vi "(FPGA)_PIDXYZ_laserPID)_COMtemp_vec_1.vi"() -> ()   [LabVIEW 2018]
doc: "This VI will read single point values from 4 channels of a R Series board at a specified rate."
uses:
  <vilib>/rvi/Emulation/niFpgaGetClockAttributes.vi
  <vilib>/rvi/Emulation/niFpgaSctlEmulationGetInTimedLoop.vi
  <vilib>/rvi/Emulation/niFpgaEmulationReportErrorSimple.vi
  <vilib>/rvi/eio/common/nirviEmuTemplateMethod_errors.vi
  <vilib>/rvi/Emulation/niFpgaProcessEmulError.vi
  <vilib>/rvi/Emulation/niFpgaCriticalErrorInLSC.vi
  <vilib>/rvi/Memory/Memory_Emulation/nirvimemoryFastEmulation.vi
  <vilib>/rvi/Memory/Memory_Emulation/nirvimemoryEmulation.vi
  <vilib>/rvi/Emulation/niFpgaEmulationIsFPGAContextNoSignature.vi
  <vilib>/rvi/DataTransferAndStorage/Container/Common/niFpgaContainerGetUniqueNameForEmu.vi
  <vilib>/rvi/errors/nirviReportUnexpectedCaseInternalError (U32).vi
  <vilib>/rvi/Memory/Memory_Emulation/niFpgaMemoryEmulationCacheClearOnFirstRun.vi
  <vilib>/rvi/Memory/Memory_Emulation/nirvimemoryEmulationManagerCache_MakeExclusive.vi
  <vilib>/rvi/Memory/Memory_Emulation/niFpgaMemoryEmulationValidateCache.vi
  <vilib>/rvi/Memory/Memory_Emulation/nirvimemoryEmulationManagerCache_InsertValue.vi
  <vilib>/Utility/error.llb/Clear Errors.vi
  <vilib>/rvi/Memory/Memory_Emulation/nirvimemoryEmulationManagerCache_ReleaseExclusive.vi
  <vilib>/rvi/Memory/Memory_Emulation/nirvimemoryEmulationManagerCache_GetValue.vi
  <vilib>/rvi/Memory/Memory_Emulation/nirvimemoryEmulationManagerCache_SetValue.vi
  <vilib>/rvi/Emulation/niFpgaSctlEmulationResourceMgr.vi
  <vilib>/eio/EIONode/EIONode.xnode
  <vilib>/rvi/DataTransferAndStorage/Container/XNode/niFpgaContainer.xnode
  <vilib>/rvi/FXPMathLib/FxpInterpret/XNode/nifxpmath_Interpret.xnode
panel:
  in  "Amplitude AO7":fxp<+/-,64,32>
  in  "Amplitude AO6":fxp<+/-,64,32>
  in  "Amplitude AO5":fxp<+/-,64,32>
  in  "Amplitude AO4":fxp<+/-,64,32>
  in  "phase offset AO7":fxp<+,32,0>
  in  "reset AO7":bool
  in  "frequency AO7":fxp<+,32,0>=0.0002500000409781933
  in  "phase offset AO6":fxp<+,32,0>
  in  "reset AO6":bool
  in  "frequency AO6":fxp<+,32,0>=0.0002500000409781933
  in  "phase offset AO5":fxp<+,32,0>
  in  "reset AO5":bool
  in  "frequency AO5":fxp<+,32,0>=0.0002500000409781933
  in  "phase offset AO4":fxp<+,32,0>
  in  "reset AO4":bool
  in  "frequency AO4":fxp<+,32,0>=0.0002500000409781933
  in  "stop":bool
  in  "Notch coeff y 2":i32[](array[numeric])=[-1060332860, 1067037342, -2129863576]
  in  "Notch coeff y 1":i32[](array[numeric])=[-1060332860, 1067037342, -2129863576]
  in  "Notch coeff x":i32[](array[numeric])=[-1060332860, 1067037342, -2129863576]
  out "accum out z2":fxp<+/-,37,37>
  out "accurm reset z2":bool
  out "accum out z1":fxp<+/-,37,37>
  out "accum reset z1":bool
  in  "Reset x accum":bool
  in  "Reset y accum":bool
  in  "Reset z accum":bool
  out "master y":bool
  out "master x":bool
  in  "No_integral_gain":bool=TRUE
  in  "Y_emergency_threshould":i16
  in  "X_emergency_threshould":i16
  in  "Big Number":sgl
  in  "Amplitude_sine_EOM":sgl
  in  "eom sine frequency (periods/tick)":fxp<+,32,0>=0.0002500000409781933
  in  "pz?":bool
  out "pg Z mod":fxp<+/-,24,12>
  in  "pg Z":fxp<+/-,24,12>
  in  "amplitude":i16=8192
  in  "offset":i16=8192
  out "Trigger for COM out":i16 caption="square wave out"
  out "dgz mod":fxp<+/-,24,12>
  in  "activate COMz":bool
  in  "dg Z":fxp<+/-,24,12>
  in  "activate COMy":bool
  out "dgy mod":fxp<+/-,24,12>
  in  "dg Y":fxp<+/-,24,12>
  out "dgx mod":fxp<+/-,24,12>
  in  "activate COMx":bool
  in  "dg X":fxp<+/-,24,12>
  in  "duty cycle (periods)":fxp<+,32,0>=0.5
  in  "frequency (periods/tick)":fxp<+,32,0>=0.00390625
  in  "final filter coeff X before":i32[](array[numeric])=[-955995012, 2025731616, 1001305, -1023351008, 2092954700, 1034533]
  in  "final filter coeff X":i32[](array[numeric])=[-955995012, 2025731616, 1001305, -1023351008, 2092954700, 1034533]
  in  "final filter coeff Y before":i32[](array[numeric])=[-955995012, 2025731616, 1001305, -1023351008, 2092954700, 1034533]
  in  "final filter coeff Y":i32[](array[numeric])=[-955995012, 2025731616, 1001305, -1023351008, 2092954700, 1034533]
  in  "final filter coeff Z":i32[](array[numeric])=[-955995012, 2025731616, 1001305, -1023351008, 2092954700, 1034533]
  in  "final filter coeff Z before":i32[](array[numeric])=[-955995012, 2025731616, 1001305, -1023351008, 2092954700, 1034533]
  in  "LP Coeff Z before":i32[](array[numeric])=[1008310688, 32715568]
  in  "LP Coeff Z":i32[](array[numeric])=[1008310688, 32715568]
  in  "LP Coeff X":i32[](array[numeric])=[1008310688, 32715568]
  in  "LP Coeff X before":i32[](array[numeric])=[1008310688, 32715568]
  in  "LP Coeff Y before":i32[](array[numeric])=[1008310688, 32715568]
  in  "LP Coeff Y":i32[](array[numeric])=[1008310688, 32715568]
  in  "Upper lim Z before":fxp<+/-,16,16>
  in  "Lower lim Z before":fxp<+/-,16,16>
  in  "Upper lim Y before":fxp<+/-,16,16>
  in  "Lower lim Y before":fxp<+/-,16,16>
  in  "Upper lim X before":fxp<+/-,16,16>
  in  "Lower lim X before":fxp<+/-,16,16>
  in  "HP coeff band X before":i32[](array[numeric])=[-850883994, 1909449570, 958518847, -975456236, 2033039520, 1020559395]
  in  "LP Coeff band X before":i32[](array[numeric])=[-955995012, 2025731616, 1001305, -1023351008, 2092954700, 1034533]
  in  "LP Coeff band X":i32[](array[numeric])=[-955995012, 2025731616, 1001305, -1023351008, 2092954700, 1034533]
  in  "HP Coeff band X":i32[](array[numeric])=[-850883994, 1909449570, 958518847, -975456236, 2033039520, 1020559395]
  in  "dg band X before":fxp<+/-,24,12>
  in  "dg band X":fxp<+/-,24,12>
  in  "HP Coeff X before":i32[](array[numeric])=[946630756, 1010186290]
  in  "HP Coeff X":i32[](array[numeric])=[946630756, 1010186290]
  in  "Use X PID before":bool
  out "AI X before chamber plot":i16
  in  "X before Setpoint":i16
  out "tot_fb X plot":i16
  out "fb X before chamber plot":i16
  in  "DC offset X":i16
  in  "pg X before":fxp<+/-,24,12>
  in  "ig X before":fxp<+/-,24,-4>
  in  "dg X before":fxp<+/-,24,12>
  out "fb X plot":i16
  in  "ig X":fxp<+/-,24,-4>
  in  "Lower lim X":fxp<+/-,16,16>
  in  "Upper lim X":fxp<+/-,16,16>
  in  "pg X":fxp<+/-,24,12>
  out "AI X plot":i16
  in  "X Setpoint":i16
  in  "HP coeff band Y before":i32[](array[numeric])=[-850883994, 1909449570, 958518847, -975456236, 2033039520, 1020559395]
  in  "LP Coeff band Y before":i32[](array[numeric])=[-955995012, 2025731616, 1001305, -1023351008, 2092954700, 1034533]
  in  "LP Coeff band Y":i32[](array[numeric])=[-955995012, 2025731616, 1001305, -1023351008, 2092954700, 1034533]
  in  "HP Coeff band Y":i32[](array[numeric])=[-850883994, 1909449570, 958518847, -975456236, 2033039520, 1020559395]
  in  "dg band Y before":fxp<+/-,24,12>
  in  "dg band Y":fxp<+/-,24,12>
  in  "HP Coeff Y before":i32[](array[numeric])=[946630756, 1010186290]
  in  "HP Coeff Y":i32[](array[numeric])=[946630756, 1010186290]
  in  "Use Y PID before":bool
  out "AI Y before chamber plot":i16
  in  "Y before Setpoint":i16
  out "tot_fb Y plot":i16
  out "fb Y before chamber plot":i16
  in  "DC offset Y":i16
  in  "pg Y before":fxp<+/-,24,12>
  in  "ig Y before":fxp<+/-,24,-4>
  in  "dg Y before":fxp<+/-,24,12>
  out "fb Y plot":i16
  in  "ig Y":fxp<+/-,24,-4>
  in  "Lower lim Y":fxp<+/-,16,16>
  in  "Upper lim Y":fxp<+/-,16,16>
  in  "pg Y":fxp<+/-,24,12>
  out "AI Y plot":i16
  in  "Y Setpoint":i16
  in  "EOM_offset":i16
  in  "EOM_seed":u32=4294967295 caption="seed"
  in  "EOM reset":bool caption="reset"
  in  "EOM_threshold":i16
  in  "EOM_amplitude":i16
  in  "HP coeff band Z before":i32[](array[numeric])=[-850883994, 1909449570, 958518847, -975456236, 2033039520, 1020559395]
  in  "LP Coeff band Z before":i32[](array[numeric])=[-955995012, 2025731616, 1001305, -1023351008, 2092954700, 1034533]
  in  "LP Coeff band Z":i32[](array[numeric])=[-955995012, 2025731616, 1001305, -1023351008, 2092954700, 1034533]
  in  "HP Coeff band Z":i32[](array[numeric])=[-850883994, 1909449570, 958518847, -975456236, 2033039520, 1020559395]
  in  "dg band Z before":fxp<+/-,24,12>
  in  "dg band Z":fxp<+/-,24,12>
  in  "data_buffer3":i16
  in  "Arb gain (ch2)":fxp<+/-,24,12>=0.5 caption="RMS"
  in  "HP Coeff Z before":i32[](array[numeric])=[946630756, 1010186290]
  in  "HP Coeff Z":i32[](array[numeric])=[946630756, 1010186290]
  in  "Use Z PID before":bool
  out "AI Z before chamber plot":i16
  in  "Z before Setpoint":i16
  out "tot_fb Z plot":i16
  out "fb Z before chamber plot":i16
  in  "DC offset Z":i16
  in  "pg Z before":fxp<+/-,24,12>
  in  "ig Z before":fxp<+/-,24,-4>
  in  "dg Z before":fxp<+/-,24,12>
  out "fb Z plot":i16
  in  "ig Z":fxp<+/-,24,-4>
  out "written_address":u32
  in  "ready_to_write":bool
  in  "Arb steps per cycle":u16
  in  "data_buffer2":i16
  in  "data_buffer_1":i16
  in  "write_address":u16
  in  "Arb gain (ch1)":fxp<+/-,24,12>=0.5 caption="RMS"
  in  "Arb gain (ch0)":fxp<+/-,24,12>=0.5 caption="RMS"
  in  "Lower lim Z":fxp<+/-,16,16>
  in  "Upper lim Z":fxp<+/-,16,16>
  out "AI Z plot":i16
  in  "Z Setpoint":i16
  in  "Count(uSec)":u32
  out "FPGA Error Out":errorcluster
  in  "Stop":bool
  # "test"
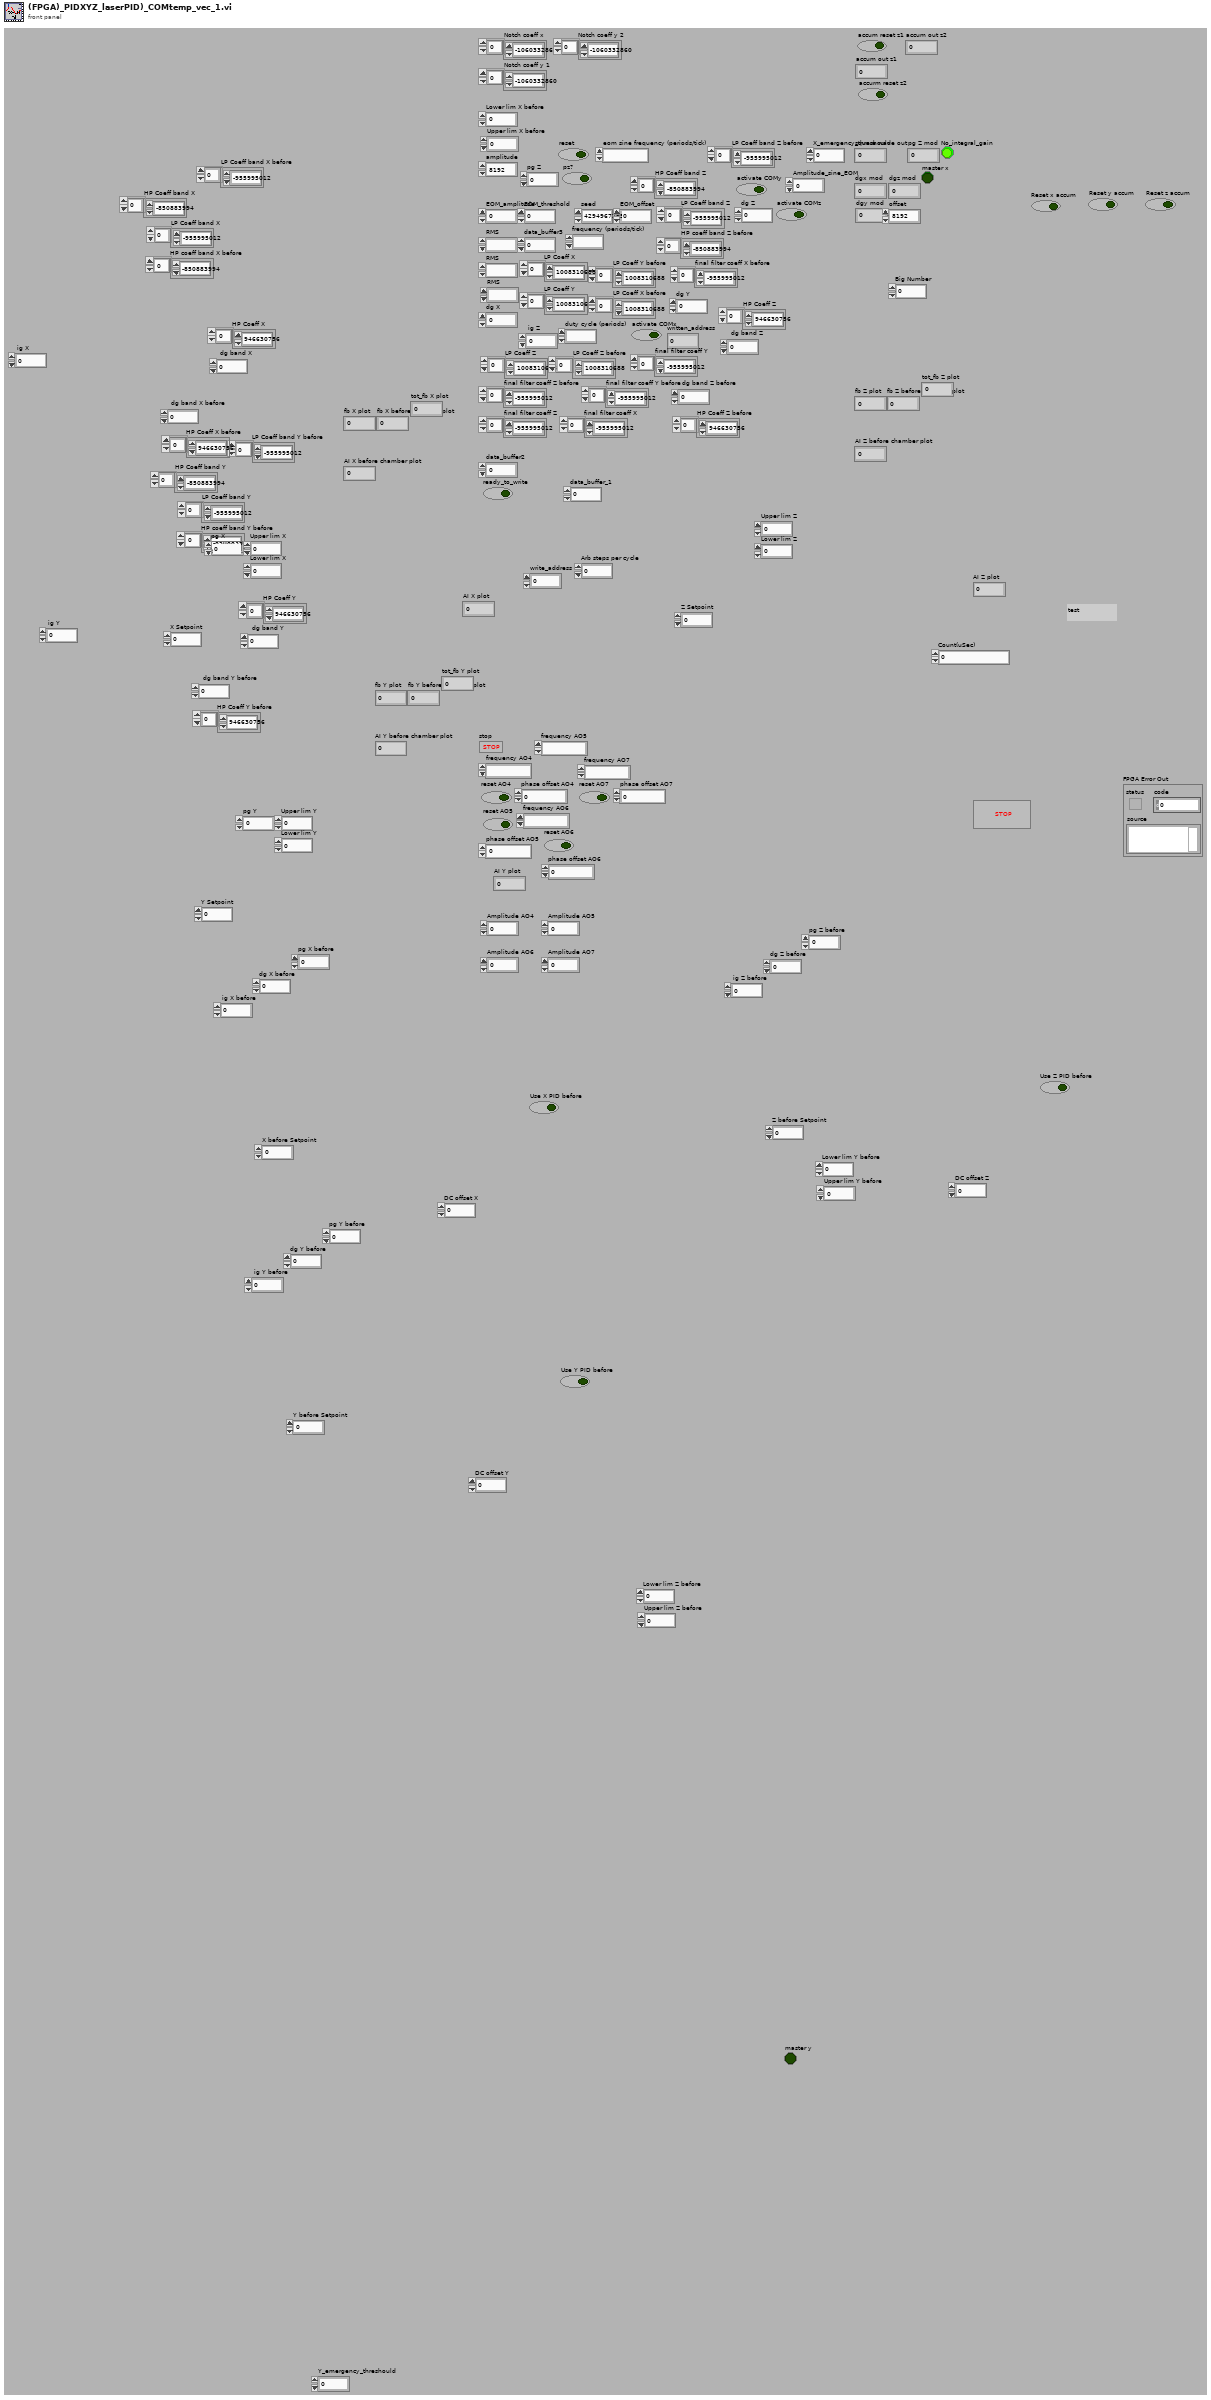
[diagram p1: front panel]
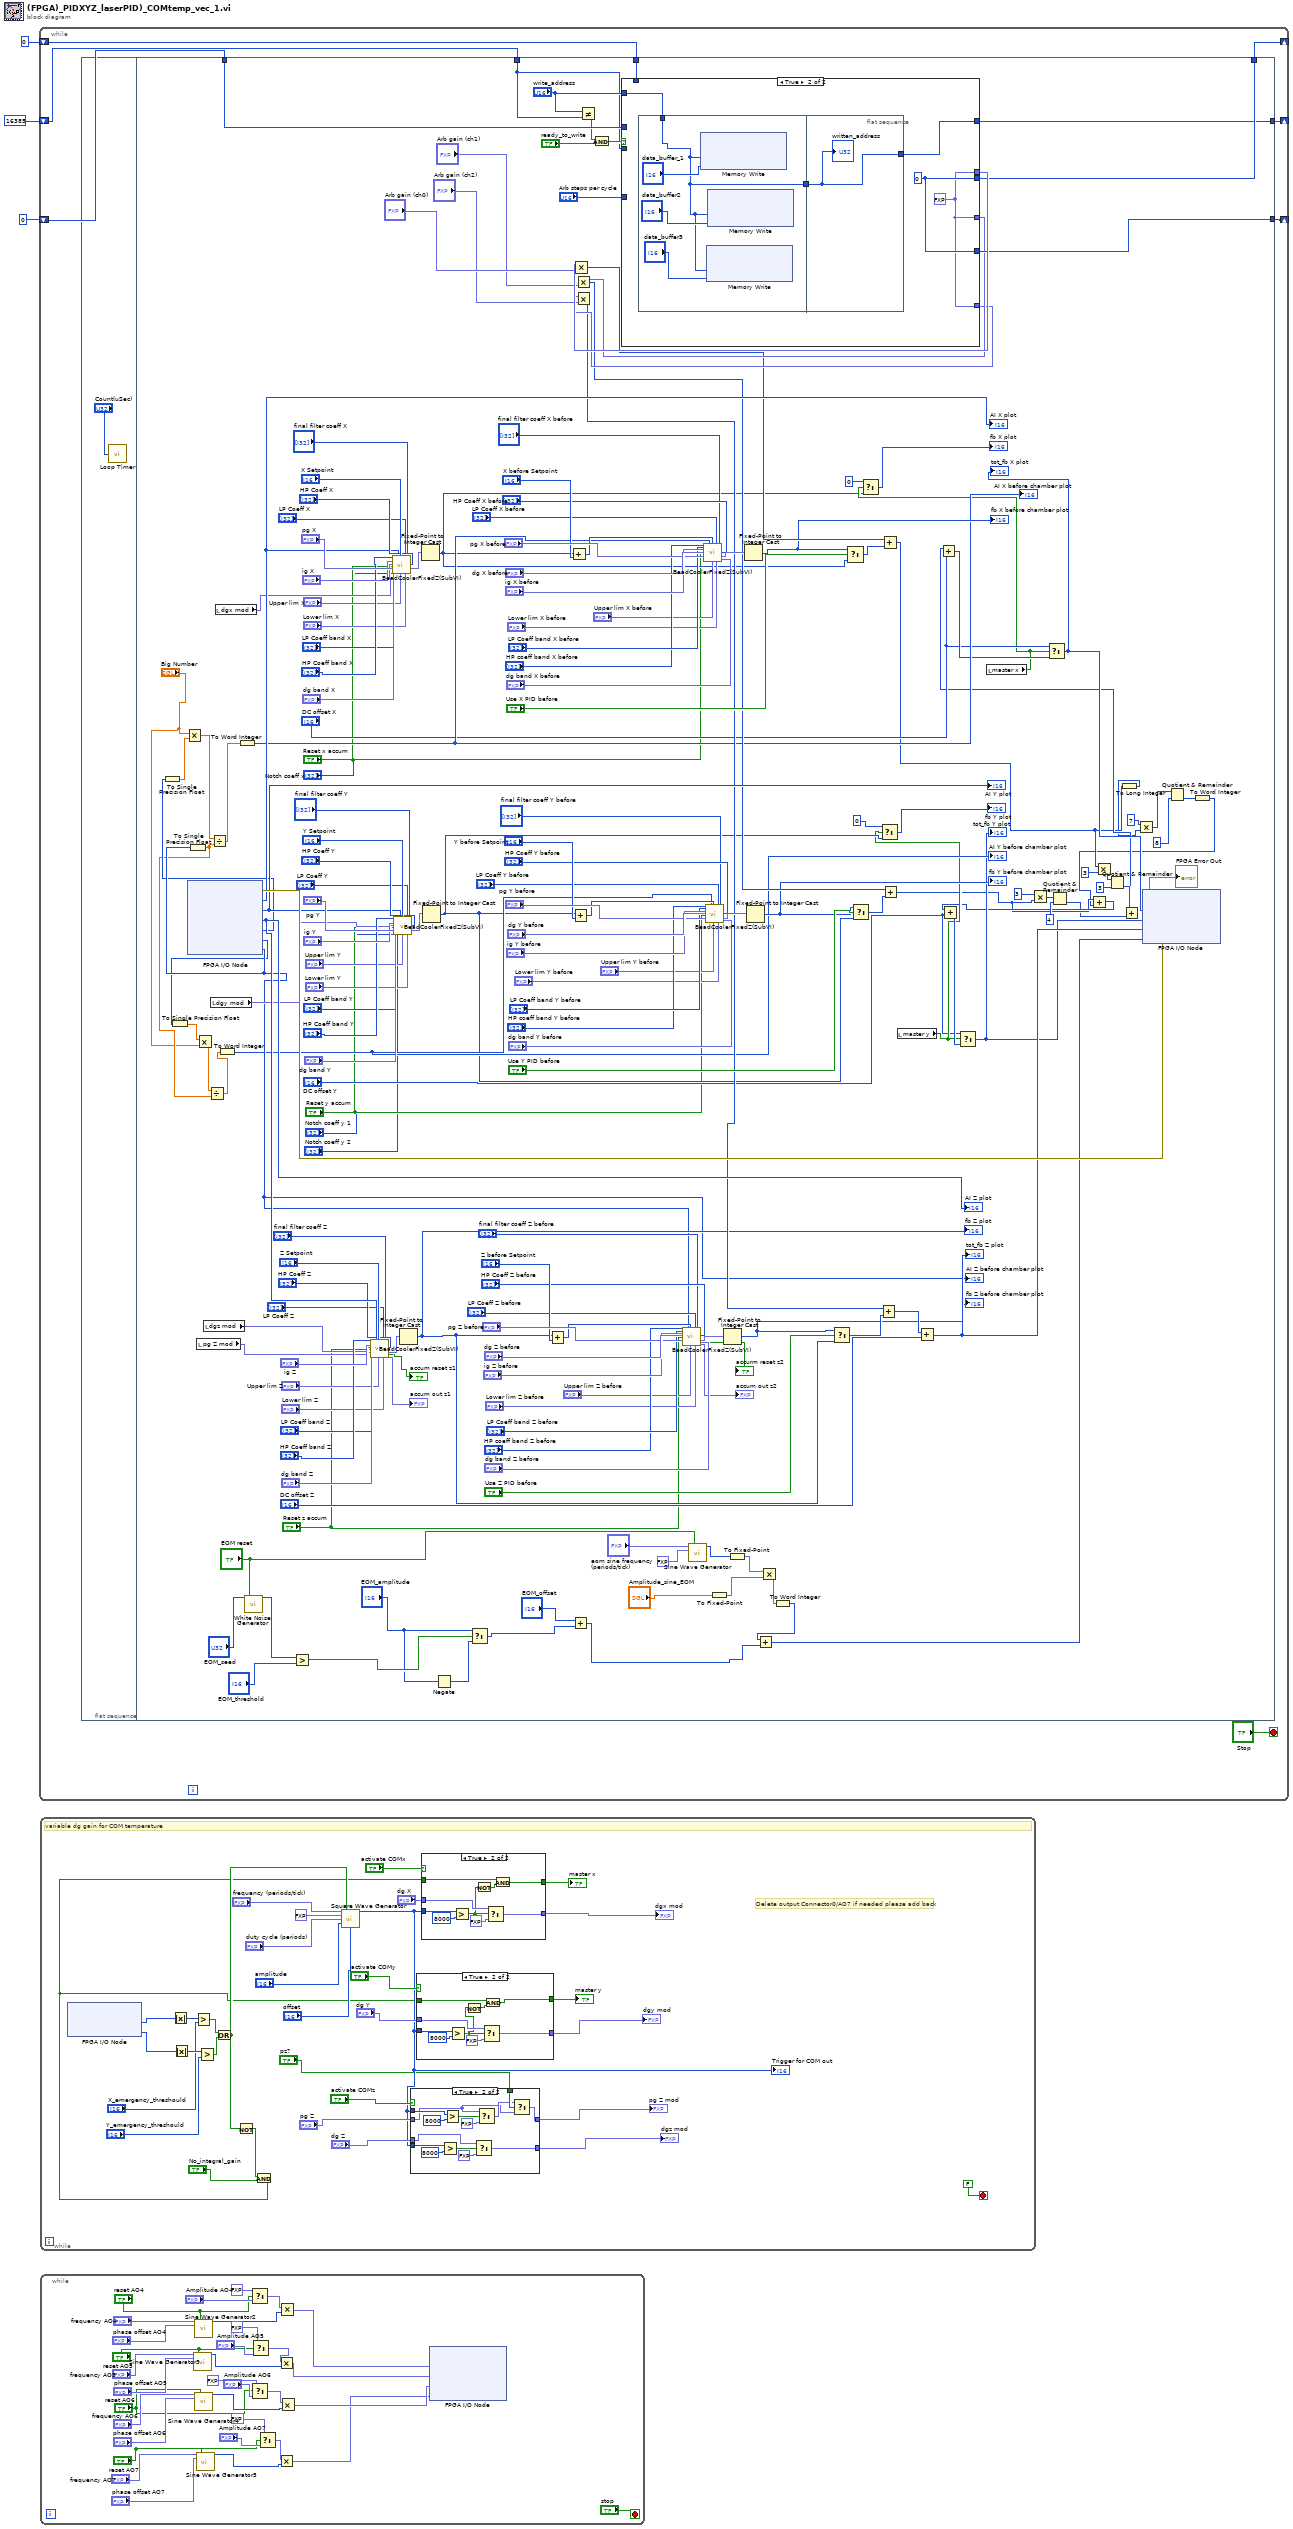
[diagram p0: block diagram]
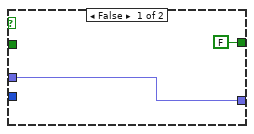
[diagram p3: hidden frame]
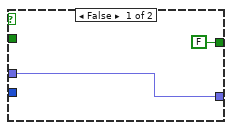
[diagram p4: hidden frame]
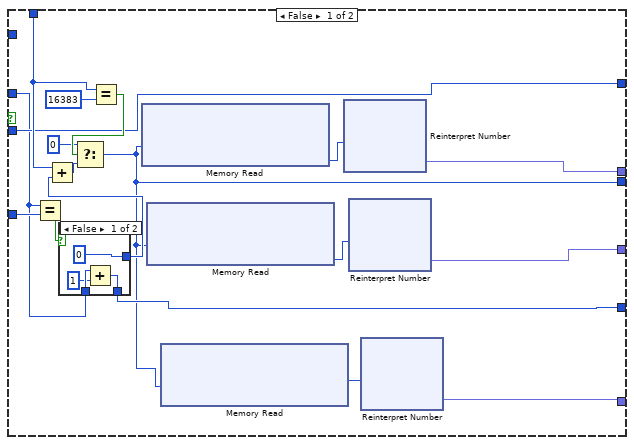
[diagram p5: hidden frame]
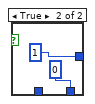
[diagram p6: hidden frame]
diagram:
  n1 = while {
    shift-right: [w9] -> _
    shift-left: u16 0 ("t") -> [w8]
    shift-right: [w7] -> _
    shift-left: u16 0 ("t") -> [w4]
    shift-right: [w6] -> _
    shift-left: u32 16385 ("write_address") -> [w5]
    stop <- "Stop" stop-if-true
    n2 = flat-sequence {
      tunnel: [w199] -> w9
      tunnel: w8 -> [w198]
      tunnel: [w196] -> w7
      tunnel: w4 -> [w195]
      tunnel: [w194] -> w6
      tunnel: w5 -> [w187]
      frame #0 {
        n3 = call "Loop Timer"("Count(uSec)"="Count(uSec)") -> ()  [unwired: 1 out]
      }
      frame #1 {
        n4 = xnode "FPGA I/O Node"() -> ("error out"=w204:errorcluster, "Connector0/AI0"=w111:i16, "Connector0/AI1"=w133:i16, "Connector0/AI2"=w185:i16, "Connector0/AI3"=w61:i16, "Connector0/AI4"=w60:i16, "Connector0/AI5"=w65:i16)  [unwired: 7 in, 6 out]
        "AI Z plot" <- w185
        "AI Z before chamber plot" <- w65
        "AI Y plot" <- w133
        "AI X plot" <- w111
        n5 = To Single Precision Float(number=w61) -> (single precision float=w64:sgl)
        n6 = To Single Precision Float(number=w60) -> (single precision float=w59:sgl)
        n7 = Multiply(x="Big Number", y=w64) -> (x*y=w63:sgl)
        n8 = To Single Precision Float(number=w65) -> (single precision float=w57:sgl)
        n9 = Multiply(x=w59, y="Big Number") -> (x*y=w58:sgl)
        n10 = local read "pg Z mod"() -> (w78:fxp<+/-,24,12>)
        n11 = local read "dgz mod"() -> (w79:fxp<+/-,24,12>)
        n12 = Divide(x=w58, y=w57) -> (x/y=w56:sgl)
        n13 = Divide(x=w63, y=w57) -> (x/y=w62:sgl)
        n14 = local read "dgy mod"() -> (w80:fxp<+/-,24,12>)
        n15 = local read "dgx mod"() -> (w81:fxp<+/-,24,12>)
        n16 = To Word Integer(number=w56) -> (16bit integer=w55:i16)
        "AI Y before chamber plot" <- w55
        n17 = To Word Integer(number=w62) -> (16bit integer=w66:i16)
        "AI X before chamber plot" <- w66
        n18 = call "White Noise Generator"("seed"="EOM_seed", "reset"="EOM reset") -> ("white noise out"=w164:i16)  [unwired: 13 in]
        n19 = Greater?(x=w164, y="EOM_threshold") -> (0:w162:bool)
        n20 = call "BeadCoolerFixedZ(SubVI).vi"("hp coeff band"="HP Coeff band Z", "lp coeff band"="LP Coeff band Z", "ig"="ig Z", "dg"=w79, "load (F)"="Reset z accum", "pg"=w78, "dg band"="dg band Z", "AI0"=w185, "Dc Pos"="Z Setpoint", "Upper lim"="Upper lim Z", "lp coeff"="LP Coeff Z", "Lower lim"="Lower lim Z", "final filter coeff"="final filter coeff Z", "hp coeff"="HP Coeff Z") -> ("Output"=w174:fxp<+/-,16,16>, "accurm reset"=→"accum reset z1":bool, "accum out"=→"accum out z1":fxp<+/-,37,37>)  [unwired: 11 in]
        n21 = call "BeadCoolerFixedZ(SubVI).vi"("hp coeff band"="HP Coeff band X", "lp coeff band"="LP Coeff band X", "ig"="ig X", "dg"=w81, "load (F)"="Reset x accum", "pg"="pg X", "dg band"="dg band X", "Notch coeff 1"="Notch coeff x", "AI0"=w111, "Dc Pos"="X Setpoint", "Upper lim"="Upper lim X", "lp coeff"="LP Coeff X", "Lower lim"="Lower lim X", "final filter coeff"="final filter coeff X", "hp coeff"="HP Coeff X") -> ("Output"=w121:fxp<+/-,16,16>)  [unwired: 10 in, 2 out]
        n22 = call "BeadCoolerFixedZ(SubVI).vi"("hp coeff band"="HP Coeff band Y", "lp coeff band"="LP Coeff band Y", "ig"="ig Y", "dg"=w80, "load (F)"="Reset y accum", "pg"="pg Y", "dg band"="dg band Y", "Notch coeff 1"="Notch coeff y 1", "Notch coeff 2"="Notch coeff y 2", "AI0"=w133, "Dc Pos"="Y Setpoint", "Upper lim"="Upper lim Y", "lp coeff"="LP Coeff Y", "Lower lim"="Lower lim Y", "final filter coeff"="final filter coeff Y", "hp coeff"="HP Coeff Y") -> ("Output"=w143:fxp<+/-,16,16>)  [unwired: 9 in, 2 out]
        n23 = Fixed-Point to Integer Cast(1:w174) -> (0:w89:i16)
        "fb Z plot" <- w89
        n24 = Fixed-Point to Integer Cast(1:w121) -> (0:w43:i16)
        n25 = Fixed-Point to Integer Cast(1:w143) -> (0:w50:i16)
        n26 = Negate(x="EOM_amplitude") -> (-x=w160:i16)
        n27 = Select(t="EOM_amplitude", s=w162, f=w160) -> (s? t:f=w158:i16)
        n28 = Add(x=w89, y="Z before Setpoint") -> (x+y=w173:i16)
        n29 = Add(x=w43, y="X before Setpoint") -> (x+y=w120:i16)
        n30 = Add(x=w50, y="Y before Setpoint") -> (x+y=w142:i16)
        n31 = Add(x="EOM_offset", y=w158) -> (x+y=w69:i16)
        n32 = Not Equal?(x="write_address", y=w187) -> (x != y?=w191:bool)
        n33 = And(x=w191, y="ready_to_write") -> (x .and. y?=w192:bool)
        n34 = case shown="True" w192 {
          tunnel: [w221 w229] -> w201
          tunnel: [w206 w233] -> w199
          tunnel: w198 -> [w214 _]
          tunnel: [w215 w229] -> w189
          tunnel: "Arb steps per cycle" -> [w213 _]
          tunnel: [w208 w233] -> w196
          tunnel: w195 -> [w209 _]
          tunnel: [w212 w231] -> w194
          tunnel: w187 -> [w212 _]
          tunnel: "write_address" -> [_ w230]
          tunnel: [w205 w229] -> w171
          frame False {
            n35 = Equal?(x=w209, y=w213) -> (x = y?=w211:bool)
            n36 = case shown="False" w211 {
              tunnel: [u16 0 ("y") u16 1 ("y")] -> w210
              tunnel: w209 -> [w225 _]
              tunnel: [w223 u16 0] -> w208
              frame False {
                n37 = Add(x=w225, y=u16 1) -> (x+y=w223:u16)
              }
              frame True {
              }
            }
            n38 = Add(x=w214, y=w210) -> (x+y=w217:u16)
            n39 = Equal?(x=w214, y=u16 16383) -> (x = y?=w219:bool)
            n40 = Select(t=u16 0, s=w219, f=w217) -> (s? t:f=w206:u16)
            n41 = xnode ("Memory Read")("Address"=w206) -> ("Data"=w222:i16)  [unwired: 1 in, 1 out]
            n42 = xnode ("Memory Read")("Address"=w206) -> ("Data"=w216:i16)  [unwired: 1 in, 1 out]
            n43 = xnode ("Memory Read")("Address"=w206) -> ("Data"=w207:i16)  [unwired: 1 in, 1 out]
            n44 = xnode "Reinterpret Number"("x"=w222) -> ("y"=w221:fxp<+/-,16,16>)
            n45 = xnode "Reinterpret Number"("x"=w216) -> ("y"=w215:fxp<+/-,16,16>)
            n46 = xnode "Reinterpret Number"("x"=w207) -> ("y"=w205:fxp<+/-,16,16>)
          }
          frame True {
            w233 = u16 0
            w229 = fxp<+/-,16,16> 0.0 ("y")
            n47 = flat-sequence {
              tunnel: [w235] -> w232
              tunnel: w230 -> [w235]
              tunnel: w232 -> [w238]
              tunnel: [w238] -> w231
              frame #0 {
                n48 = xnode ("Memory Write")("Address"=w235, "Data"="data_buffer_1") -> ()  [unwired: 1 in, 1 out]
                n49 = xnode ("Memory Write")("Address"=w235, "Data"="data_buffer3") -> ()  [unwired: 1 in, 1 out]
                n50 = xnode ("Memory Write")("Address"=w235, "Data"="data_buffer2") -> ()  [unwired: 1 in, 1 out]
              }
              frame #1 {
                "written_address" <- w238
              }
            }
          }
        }
        n51 = Multiply(x=w201, y="Arb gain (ch0)") -> (x*y=w92:i16)
        n52 = Multiply(x=w189, y="Arb gain (ch1)") -> (x*y=w91:i16)
        n53 = Multiply(x=w171, y="Arb gain (ch2)") -> (x*y=w90:i16)
        n54 = call "BeadCoolerFixedZ(SubVI).vi"("hp coeff band"="HP coeff band Z before", "lp coeff band"="LP Coeff band Z before", "ig"="ig Z before", "dg"="dg Z before", "load (F)"="Reset z accum", "pg"="pg Z before", "dg band"="dg band Z before", "AI0"=w65, "Dc Pos"=w173, "Upper lim"="Upper lim Z before", "lp coeff"="LP Coeff Z before", "Lower lim"="Lower lim Z before", "final filter coeff"="final filter coeff Z before", "hp coeff"="HP Coeff Z before") -> ("Output"=w181:fxp<+/-,16,16>, "accurm reset"=→"accurm reset z2":bool, "accum out"=→"accum out z2":fxp<+/-,37,37>)  [unwired: 11 in]
        n55 = call "Sine Wave Generator"("frequency (periods/tick)"="eom sine frequency (periods/tick)", "reset"="EOM reset", "phase offset (periods)"=fxp<+,32,0> 0.0) -> ("sine out"=w75:i16)  [unwired: 12 in]
        n56 = call "BeadCoolerFixedZ(SubVI).vi"("hp coeff band"="HP coeff band X before", "lp coeff band"="LP Coeff band X before", "ig"="ig X before", "dg"="dg X before", "load (F)"="Reset x accum", "pg"="pg X before", "dg band"="dg band X before", "AI0"=w66, "Dc Pos"=w120, "Upper lim"="Upper lim X before", "lp coeff"="LP Coeff X before", "Lower lim"="Lower lim X before", "final filter coeff"="final filter coeff X before", "hp coeff"="HP Coeff X before") -> ("Output"=w126:fxp<+/-,16,16>)  [unwired: 11 in, 2 out]
        n57 = call "BeadCoolerFixedZ(SubVI).vi"("hp coeff band"="HP coeff band Y before", "lp coeff band"="LP Coeff band Y before", "ig"="ig Y before", "dg"="dg Y before", "load (F)"="Reset y accum", "pg"="pg Y before", "dg band"="dg band Y before", "AI0"=w55, "Dc Pos"=w142, "Upper lim"="Upper lim Y before", "lp coeff"="LP Coeff Y before", "Lower lim"="Lower lim Y before", "final filter coeff"="final filter coeff Y before", "hp coeff"="HP Coeff Y before") -> ("Output"=w148:fxp<+/-,16,16>)  [unwired: 11 in, 2 out]
        n58 = To Fixed-Point(number="Amplitude_sine_EOM") -> (fixed-point=w73:fxp<+/-,32,16>)  [unwired: 1 in]
        n59 = Fixed-Point to Integer Cast(1:w181) -> (0:w82:i16)
        "fb Z before chamber plot" <- w82
        n60 = To Fixed-Point(number=w75) -> (fixed-point=w74:fxp<+/-,16,16>)  [unwired: 1 in]
        n61 = Fixed-Point to Integer Cast(1:w126) -> (0:w87:i16)
        "fb X before chamber plot" <- w87
        n62 = Fixed-Point to Integer Cast(1:w148) -> (0:w85:i16)
        "fb Y before chamber plot" <- w85
        n63 = Multiply(x=w74, y=w73) -> (x*y=w72:fxp<+/-,48,32>)
        n64 = To Word Integer(number=w72) -> (16bit integer=w70:i16)
        n65 = Add(x=w70, y=w69) -> (x+y=w68:i16)
        n66 = Select(t=w82, s="Use Z PID before", f=w89) -> (s? t:f=w84:i16)
        n67 = Select(t=w87, s="Use X PID before", f=w43) -> (s? t:f=w88:i16)
        n68 = Select(t=w85, s="Use Y PID before", f=w50) -> (s? t:f=w86:i16)
        n69 = Add(x=w90, y=w84) -> (x+y=w83:i16)
        n70 = Add(x=w92, y=w88) -> (x+y=w15:i16)
        n71 = Add(x=w91, y=w86) -> (x+y=w17:i16)
        n72 = local read "master y"() -> (w49:bool)
        n73 = Select(t=i16 0, s=w49, f=w50) -> (s? t:f=→"fb Y plot":i16)
        n74 = Add(x=w83, y="DC offset Z") -> (x+y=w177:i16)
        "tot_fb Z plot" <- w177
        n75 = local read "master x"() -> (w45:bool)
        n76 = Select(t=i16 0, s=w45, f=w43) -> (s? t:f=→"fb X plot":i16)
        n77 = Multiply(x=i16 3, y=w17) -> (x*y=w26:i16)
        n78 = Quotient & Remainder(x=w26, y=i16 4 ("x")) -> (floor(x/y)=w16:i16)  [unwired: 1 out]
        n79 = Multiply(x=w15, y=i16 3 ("x")) -> (x*y=w22:i16)
        n80 = Quotient & Remainder(x=w22, y=i16 3 ("x")) -> (floor(x/y)=w19:i16)  [unwired: 1 out]
        n81 = To Long Integer(number=w15) -> (32bit integer=w14:i32)
        n82 = Add(x=w19, y=w16) -> (x+y=w18:i16)
        n83 = Add(x=w18, y="DC offset X") -> (x+y=w47:i16)
        n84 = Select(t="DC offset X", s=w45, f=w47) -> (s? t:f=w23:i16)
        "tot_fb X plot" <- w23
        n85 = Multiply(x=i16 7, y=w14) -> (x*y=w27:i32)
        n86 = Quotient & Remainder(x=w27, y=i16 8 ("x")) -> (floor(x/y)=w13:i32)  [unwired: 1 out]
        n87 = To Word Integer(number=w13) -> (16bit integer=w12:i16)
        n88 = Add(x=w17, y=w12) -> (x+y=w21:i16)
        n89 = Add(x=w21, y="DC offset Y") -> (x+y=w53:i16)
        n90 = Select(t="DC offset Y", s=w49, f=w53) -> (s? t:f=w24:i16)
        "tot_fb Y plot" <- w24
        n91 = xnode "FPGA I/O Node"("error in"=w204, "Connector0/AO0"=w23, "Connector0/AO1"=w24, "Connector0/AO2"=w177, "Connector0/AO3"=w68) -> ("error out"=→"FPGA Error Out":errorcluster)  [unwired: 4 in, 4 out]
      }
    }
  }
  n92 = while {
    stop <- FALSE stop-if-true
    # "Delete output Connector0/AO7 if needed please add back"
    # "variable dg gain for COM temperature"
    n93 = xnode "FPGA I/O Node"() -> ("Connector0/AI0"=w252:i16, "Connector0/AI1"=w251:i16)  [unwired: 3 in, 3 out]
    n94 = Absolute Value(x=w252) -> (abs(x)=w250:i16)
    n95 = Absolute Value(x=w251) -> (abs(x)=w249:i16)
    n96 = Greater?(x=w250, y="X_emergency_threshould") -> (0:w246:bool)
    n97 = Greater?(x=w249, y="Y_emergency_threshould") -> (0:w245:bool)
    n98 = Or(x=w246, y=w245) -> (x .or. y?=w244:bool)
    n99 = Not(x=w244) -> (.not. x?=w243:bool)
    n100 = And(x=w243, y="No_integral_gain") -> (x .and. y?=w241:bool)
    n101 = call "Square Wave Generator"("frequency (periods/tick)"="frequency (periods/tick)", "reset"=w244, "phase offset (periods)"=fxp<+,32,0> 0.0, "duty cycle (periods)"="duty cycle (periods)", "amplitude"="amplitude", "offset"="offset") -> ("square wave out"=w254:i16)  [unwired: 9 in]
    "Trigger for COM out" <- w254
    n102 = case shown="True" "activate COMz" {
      tunnel: [w273 w284] -> w257
      tunnel: w254 -> [_ w287]
      tunnel: "dg Z" -> [w273 w282]
      tunnel: "pg Z" -> [w272 w274]
      tunnel: [w272 w275] -> w255
      tunnel: w254 -> [_ w278]
      tunnel: "pz?" -> [_ w277]
      frame False {
      }
      frame True {
        n103 = Greater?(x=w287, y=i16 8000) -> (0:w285:bool)
        n104 = Greater?(x=w278, y=i16 8000) -> (0:w280:bool)
        n105 = Select(t=w282, s=w285, f=fxp<+/-,24,12> 0.0 ("y")) -> (s? t:f=w284:fxp<+/-,24,12>)
        n106 = Select(t=w274, s=w280, f=fxp<+/-,24,12> 0.0 ("y")) -> (s? t:f=w276:fxp<+/-,24,12>)
        n107 = Select(t=w276, s=w277, f=w274) -> (s? t:f=w275:fxp<+/-,24,12>)
      }
    }
    "dgz mod" <- w257
    "pg Z mod" <- w255
    n108 = case shown="True" "activate COMy" {
      tunnel: "dg Y" -> [w289 w295]
      tunnel: [w289 w296] -> w261
      tunnel: w254 -> [_ w298]
      tunnel: w241 -> [_ w292]
      tunnel: [FALSE w290] -> w239
      frame False {
      }
      frame True {
        n109 = Greater?(x=w298, y=i16 8000) -> (0:w291:bool)
        n110 = Not(x=w291) -> (.not. x?=w293:bool)
        n111 = Select(t=w295, s=w291, f=fxp<+/-,24,12> 0.0 ("y")) -> (s? t:f=w296:fxp<+/-,24,12>)
        n112 = And(x=w292, y=w293) -> (x .and. y?=w290:bool)
      }
    }
    "dgy mod" <- w261
    "master y" <- w239
    n113 = case shown="True" "activate COMx" {
      tunnel: "dg X" -> [w300 w306]
      tunnel: [w300 w307] -> w263
      tunnel: w254 -> [_ w309]
      tunnel: w241 -> [_ w302]
      tunnel: [FALSE w301] -> w240
      frame False {
      }
      frame True {
        n114 = Greater?(x=w309, y=i16 8000) -> (0:w304:bool)
        n115 = Not(x=w304) -> (.not. x?=w303:bool)
        n116 = Select(t=w306, s=w304, f=fxp<+/-,24,12> 0.0 ("y")) -> (s? t:f=w307:fxp<+/-,24,12>)
        n117 = And(x=w302, y=w303) -> (x .and. y?=w301:bool)
      }
    }
    "dgx mod" <- w263
    "master x" <- w240
  }
  n118 = while {
    stop <- "stop" stop-if-true
    n119 = call "Sine Wave Generator3"("frequency (periods/tick)"="frequency AO5", "reset"="reset AO5", "phase offset (periods)"="phase offset AO5") -> ("sine out"=w331:i16)  [unwired: 12 in]
    n120 = call "Sine Wave Generator2"("frequency (periods/tick)"="frequency AO4", "reset"="reset AO4", "phase offset (periods)"="phase offset AO4") -> ("sine out"=w333:i16)  [unwired: 12 in]
    n121 = call "Sine Wave Generator4"("frequency (periods/tick)"="frequency AO6", "reset"="reset AO6", "phase offset (periods)"="phase offset AO6") -> ("sine out"=w329:i16)  [unwired: 12 in]
    n122 = call "Sine Wave Generator5"("frequency (periods/tick)"="frequency AO7", "reset"="reset AO7", "phase offset (periods)"="phase offset AO7") -> ("sine out"=w327:i16)  [unwired: 12 in]
    n123 = Select(t=fxp<+/-,64,32> 0.0, s="reset AO4", f="Amplitude AO4") -> (s? t:f=w310:fxp<+/-,64,32>)
    n124 = Select(t=fxp<+/-,64,32> 0.0, s="reset AO6", f="Amplitude AO6") -> (s? t:f=w315:fxp<+/-,64,32>)
    n125 = Select(t=fxp<+/-,64,32> 0.0, s="reset AO5", f="Amplitude AO5") -> (s? t:f=w319:fxp<+/-,64,32>)
    n126 = Select(t=fxp<+/-,64,32> 0.0, s="reset AO7", f="Amplitude AO7") -> (s? t:f=w311:fxp<+/-,64,32>)
    n127 = Multiply(x=w319, y=w331) -> (x*y=w330:fxp<+/-,64,48>)
    n128 = Multiply(x=w311, y=w327) -> (x*y=w326:fxp<+/-,64,48>)
    n129 = Multiply(x=w310, y=w333) -> (x*y=w332:fxp<+/-,64,48>)
    n130 = Multiply(x=w315, y=w329) -> (x*y=w328:fxp<+/-,64,48>)
    n131 = xnode "FPGA I/O Node"("Connector0/AO4"=w332, "Connector0/AO5"=w330, "Connector0/AO6"=w328, "Connector0/AO7"=w326) -> ()  [unwired: 5 in, 5 out]
  }
